vi "Process.vi"(8 "error in":errorcluster, 11 "Plugin in":refnum<class "Configure Visa Device Channels.lvclass">) -> (0 "error out":errorcluster, 3 "Plugin out":refnum<class "Configure Visa Device Channels.lvclass">)   [LabVIEW 2026, in "Configure Visa Device Channels.lvlib" / "Configure Visa Device Channels.lvclass"]
uses:
  Configure Visa Device Channels.lvclass
  C:/Program Files/National Instruments/LabVIEW 2026/vi.lib/FlexLogger/SDK/PluginSDK.lvlibp/PEFClasses/SDK/Plugin/Plugin.lvclass
  Configure Visa Device Channels.lvclass/Configure Visa Device Channels.ctl
  <vilib>/FlexLogger/SDK/PluginSDK.lvlibp/PEFClasses/SDK/Channel/ParameterAccess/Read String.vi
  <vilib>/FlexLogger/SDK/PluginSDK.lvlibp/PEFClasses/SDK/Channel/ParameterAccess/Read DBL.vi
  <vilib>/FlexLogger/SDK/PluginSDK.lvlibp/PEFClasses/SDK/Plugin/DataHelpers/Write 1D DBL (NChan 1Sample).vi
  C:/Program Files/National Instruments/LabVIEW 2026/vi.lib/FlexLogger/SDK/PluginSDK.lvlibp/PEFClasses/SDK/Processing Element/Processing Element.lvclass
  C:/Users/mpetrovi/OneDrive - Emerson/Documents/LabVIEW Projects/FlexLogger IO Plug-ins/Configure Visa Device Channels/Configure Visa Device Channels.lvclass
  <vilib>/FlexLogger/SDK/PluginSDK.lvlibp/PEFClasses/SDK/Plugin/Plugin.lvclass
  <vilib>/FlexLogger/SDK/PluginSDK.lvlibp/PEFClasses/SDK/Channel/Channel.lvclass
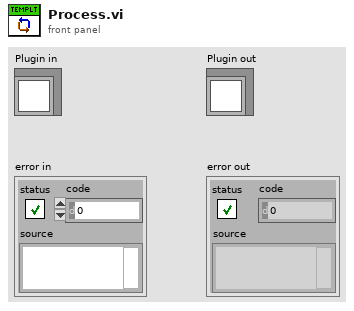
[diagram p1: front panel]
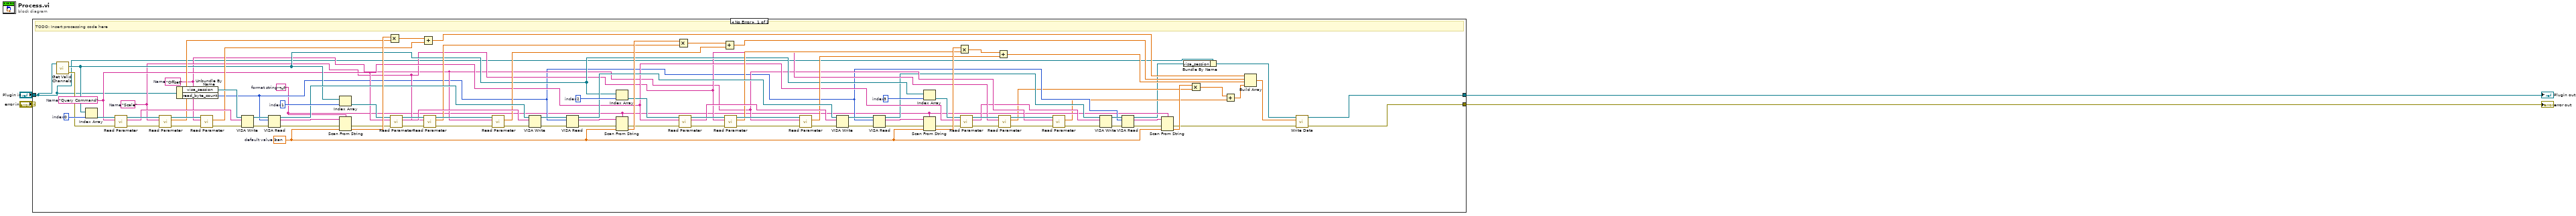
[diagram p0: block diagram]
diagram:
  n1 = case shown="No Error" "error in" {
    selector: "error in" -> [_ w95]
    tunnel: [w6 w96] -> w4
    tunnel: "Plugin in" -> [w10 w96]
    tunnel: [w5 w95] -> w1
    frame No Error {
      w39 = 3  # index
      w58 = 2  # index
      w76 = 1  # index
      w20 = "%f"  # format string
      w21 = nan  # default value 1
      w31 = "Offset"  # Name
      w34 = "Scale"  # Name
      w37 = "Query Command"  # Name
      w94 = 0  # index
      # "TODO: Insert processing code here"
      n2 = call <vilib>:"Get Valid Channels.vi"("Plugin in"=w10) -> ("error out"=w92:errorcluster, "Channels"=w40:refnum<class "Channel.lvclass">[])  [unwired: 8 in, 1 out]
      n3 = Index Array(array=w40, index=w94) -> (element=w93:refnum<class "Channel.lvclass">)
      n4 = call-poly <vilib>:"Read Parameter.vi"("error in (no error)"=w92, "Name"=w37, "Channel in"=w93) -> ("error out"=w90:errorcluster, "Value"=w86:string, "Channel out"=w91:refnum<class "Channel.lvclass">)  [unwired: 5 in, 1 out]
      n5 = call-poly <vilib>:"Read Parameter.vi"("error in (no error)"=w90, "Name"=w34, "Channel in"=w91) -> ("error out"=w88:errorcluster, "Value"=w79:dbl, "Channel out"=w89:refnum<class "Channel.lvclass">)  [unwired: 5 in, 1 out]
      n6 = Unbundle By Name(w10) -> ("visa_session"=w87:refnum<visa-resource-name>, "read_byte_count"=w25:i32)
      n7 = call-poly <vilib>:"Read Parameter.vi"("error in (no error)"=w88, "Name"=w31, "Channel in"=w89) -> ("error out"=w85:errorcluster, "Value"=w77:dbl)  [unwired: 5 in, 2 out]
      n8 = VISA Write(VISA resource name=w87, write buffer=w86, error in (no error)=w85) -> (VISA resource name out=w84:refnum<visa-resource-name>, error out=w83:errorcluster)  [unwired: 1 out]
      n9 = VISA Read(VISA resource name=w84, byte count=w25, error in (no error)=w83) -> (VISA resource name out=w69:refnum<visa-resource-name>, read buffer=w82:string, error out=w81:errorcluster)  [unwired: 1 out]
      n10 = Index Array(array=w40, index=w76) -> (element=w75:refnum<class "Channel.lvclass">)
      n11 = Scan From String(format string=w20, input string=w82, error in=w81, default 1=w21) -> (error out=w74:errorcluster, output 1=w80:dbl)  [unwired: 1 in, 2 out]
      n12 = Multiply(x=w80, y=w79) -> (x*y=w78:dbl)
      n13 = call-poly <vilib>:"Read Parameter.vi"("error in (no error)"=w74, "Name"=w37, "Channel in"=w75) -> ("error out"=w72:errorcluster, "Value"=w68:string, "Channel out"=w73:refnum<class "Channel.lvclass">)  [unwired: 5 in, 1 out]
      n14 = Add(x=w78, y=w77) -> (x+y=w15:dbl)
      n15 = call-poly <vilib>:"Read Parameter.vi"("error in (no error)"=w72, "Name"=w34, "Channel in"=w73) -> ("error out"=w70:errorcluster, "Value"=w61:dbl, "Channel out"=w71:refnum<class "Channel.lvclass">)  [unwired: 5 in, 1 out]
      n16 = call-poly <vilib>:"Read Parameter.vi"("error in (no error)"=w70, "Name"=w31, "Channel in"=w71) -> ("error out"=w67:errorcluster, "Value"=w59:dbl)  [unwired: 5 in, 2 out]
      n17 = VISA Write(VISA resource name=w69, write buffer=w68, error in (no error)=w67) -> (VISA resource name out=w66:refnum<visa-resource-name>, error out=w65:errorcluster)  [unwired: 1 out]
      n18 = VISA Read(VISA resource name=w66, byte count=w25, error in (no error)=w65) -> (VISA resource name out=w51:refnum<visa-resource-name>, read buffer=w64:string, error out=w63:errorcluster)  [unwired: 1 out]
      n19 = Index Array(array=w40, index=w58) -> (element=w57:refnum<class "Channel.lvclass">)
      n20 = Scan From String(format string=w20, input string=w64, error in=w63, default 1=w21) -> (error out=w56:errorcluster, output 1=w62:dbl)  [unwired: 1 in, 2 out]
      n21 = Multiply(x=w62, y=w61) -> (x*y=w60:dbl)
      n22 = call-poly <vilib>:"Read Parameter.vi"("error in (no error)"=w56, "Name"=w37, "Channel in"=w57) -> ("error out"=w54:errorcluster, "Value"=w50:string, "Channel out"=w55:refnum<class "Channel.lvclass">)  [unwired: 5 in, 1 out]
      n23 = Add(x=w60, y=w59) -> (x+y=w14:dbl)
      n24 = call-poly <vilib>:"Read Parameter.vi"("error in (no error)"=w54, "Name"=w34, "Channel in"=w55) -> ("error out"=w52:errorcluster, "Value"=w43:dbl, "Channel out"=w53:refnum<class "Channel.lvclass">)  [unwired: 5 in, 1 out]
      n25 = call-poly <vilib>:"Read Parameter.vi"("error in (no error)"=w52, "Name"=w31, "Channel in"=w53) -> ("error out"=w49:errorcluster, "Value"=w41:dbl)  [unwired: 5 in, 2 out]
      n26 = VISA Write(VISA resource name=w51, write buffer=w50, error in (no error)=w49) -> (VISA resource name out=w48:refnum<visa-resource-name>, error out=w47:errorcluster)  [unwired: 1 out]
      n27 = VISA Read(VISA resource name=w48, byte count=w25, error in (no error)=w47) -> (VISA resource name out=w29:refnum<visa-resource-name>, read buffer=w46:string, error out=w45:errorcluster)  [unwired: 1 out]
      n28 = Index Array(array=w40, index=w39) -> (element=w38:refnum<class "Channel.lvclass">)
      n29 = Scan From String(format string=w20, input string=w46, error in=w45, default 1=w21) -> (error out=w36:errorcluster, output 1=w44:dbl)  [unwired: 1 in, 2 out]
      n30 = Multiply(x=w44, y=w43) -> (x*y=w42:dbl)
      n31 = call-poly <vilib>:"Read Parameter.vi"("error in (no error)"=w36, "Name"=w37, "Channel in"=w38) -> ("error out"=w33:errorcluster, "Value"=w28:string, "Channel out"=w35:refnum<class "Channel.lvclass">)  [unwired: 5 in, 1 out]
      n32 = Add(x=w42, y=w41) -> (x+y=w13:dbl)
      n33 = call-poly <vilib>:"Read Parameter.vi"("error in (no error)"=w33, "Name"=w34, "Channel in"=w35) -> ("error out"=w30:errorcluster, "Value"=w18:dbl, "Channel out"=w32:refnum<class "Channel.lvclass">)  [unwired: 5 in, 1 out]
      n34 = call-poly <vilib>:"Read Parameter.vi"("error in (no error)"=w30, "Name"=w31, "Channel in"=w32) -> ("error out"=w27:errorcluster, "Value"=w16:dbl)  [unwired: 5 in, 2 out]
      n35 = VISA Write(VISA resource name=w29, write buffer=w28, error in (no error)=w27) -> (VISA resource name out=w26:refnum<visa-resource-name>, error out=w24:errorcluster)  [unwired: 1 out]
      n36 = VISA Read(VISA resource name=w26, byte count=w25, error in (no error)=w24) -> (VISA resource name out=w11:refnum<visa-resource-name>, read buffer=w23:string, error out=w22:errorcluster)  [unwired: 1 out]
      n37 = Scan From String(format string=w20, input string=w23, error in=w22, default 1=w21) -> (error out=w7:errorcluster, output 1=w19:dbl)  [unwired: 1 in, 2 out]
      n38 = Bundle By Name(cluster=w10, "visa_session"=w11) -> (w9:refnum<class "Configure Visa Device Channels.lvclass">)
      n39 = Multiply(x=w19, y=w18) -> (x*y=w17:dbl)
      n40 = Add(x=w17, y=w16) -> (x+y=w12:dbl)
      n41 = Build Array(w15, w14, w13, w12) -> (w8:dbl[])
      n42 = call-poly <vilib>:"Write Data.vi"("error in (no error)"=w7, "Data"=w8, "Plugin in"=w9) -> ("error out"=w5:errorcluster, "Plugin out"=w6:refnum<class "Configure Visa Device Channels.lvclass">)  [unwired: 7 in]
    }
    frame Error {
    }
  }
  "error out" <- w1
  "Plugin out" <- w4
